vi "Set State Machine.vi"(8 "error in (no error)":errorcluster, 11 "Channel in":refnum<class "Channel.lvclass">) -> (0 "error out":errorcluster, 3 "Channel out":refnum<class "Channel.lvclass">)   [LabVIEW 2018, in "Channel.lvclass"]
uses:
  Channel.lvclass
  Channel.lvclass/Channel.ctl
  State Machine/State Machine.lvclass
  RxTx/RxTx.lvclass
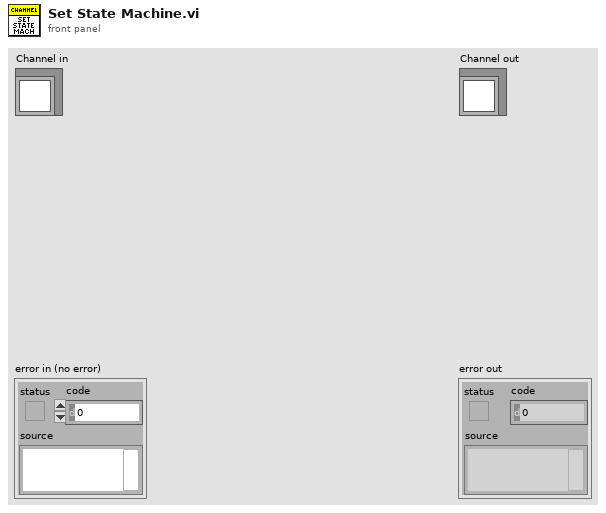
[diagram p1: front panel]
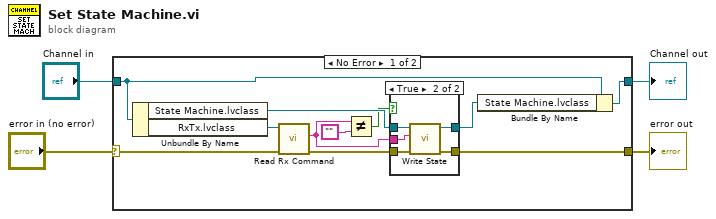
[diagram p0: block diagram]
diagram:
  n1 = case shown="No Error" "error in (no error)" {
    selector: "error in (no error)" -> [w15 w24]
    tunnel: [w9 w24] -> w3
    tunnel: [w8 w23] -> w1
    tunnel: "Channel in" -> [w11 w23]
    frame No Error {
      n2 = Unbundle By Name(w11) -> ("State Machine.lvclass"=w13:refnum<class "State Machine.lvclass">, "RxTx.lvclass"=w14:refnum<class "RxTx.lvclass">)
      n3 = call "Read Rx Command.vi"("error in (no error)"=w15, "RxTx in"=w14) -> ("error out"=w12:errorcluster, "Rx Command"=w5:string)  [unwired: 7 in, 1 out]
      n4 = Not Equal?(x=w5, y="") -> (x != y?=w7:bool)
      n5 = case shown="True" w7 {
        tunnel: w13 -> [w17 w22]
        tunnel: w12 -> [w16 w21]
        tunnel: [w17 w20] -> w10
        tunnel: [w16 w19] -> w9
        tunnel: w5 -> [_ w18]
        frame False {
        }
        frame True {
          n6 = call-dynamic "Write State.vi"("error in (no error)"=w21, "State"=w18, "State Machine in"=w22) -> ("error out"=w19:errorcluster, "State Machine out"=w20:refnum<class "State Machine.lvclass">)  [unwired: 7 in]
        }
      }
      n7 = Bundle By Name(cluster=w11, "State Machine.lvclass"=w10) -> (w8:refnum<class "Channel.lvclass">)
    }
    frame Error {
    }
  }
  "error out" <- w3
  "Channel out" <- w1
